vi "Datasocket（上课 主）.vi"() -> ()   [LabVIEW 2017]
uses:
  <vilib>/Analysis/NI_AALBase.lvlib
panel:
  in  "等待时间（毫秒）":u32=10
  out "输出簇":T1
  out "波形图":dbl[](graph)
  in  "停止":bool
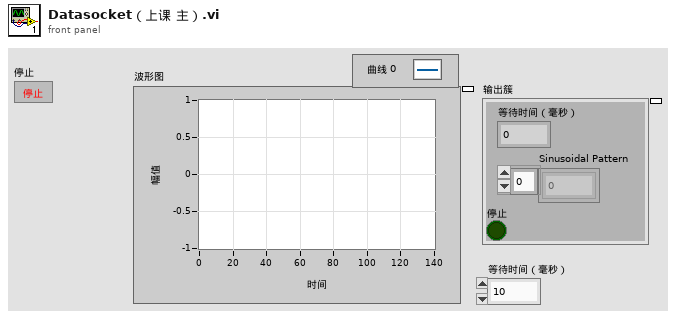
[diagram p1: front panel]
types:
  T1 = cluster{"等待时间（毫秒）":u32, "Sinusoidal Pattern":dbl[], "停止":bool}
  T2 = enum16{"Read", "Write", "ReadWrite", "BufferedRead", "BufferedReadWrite"}
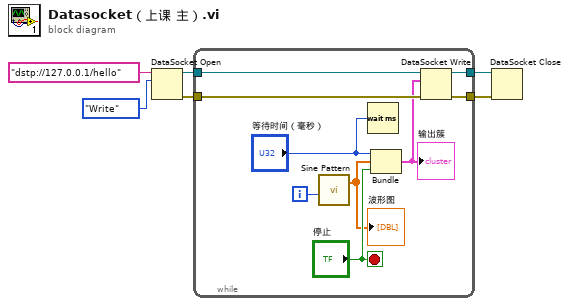
[diagram p0: block diagram]
diagram:
  n1 = DataSocket Open(10:T2."Write" ("模式"), 11:"dstp://127.0.0.1/hello" ("URL")) -> (0:w5:errorcluster, 3:w6:refnum<k13>)  [unwired: 2 in]
  n2 = while {
    tunnel: w6 -> [w11]
    tunnel: w5 -> [w10]
    tunnel: [w8] -> w3
    tunnel: [w7] -> w2
    i -> [w15]
    stop <- "停止" stop-if-true
    n3 = call <vilib>:"Sine Pattern.vi"("phase(degrees)"=w15) -> ("Sinusoidal Pattern"=w13:dbl[])  [unwired: 3 in, 1 out]
    "波形图" <- w13
    n4 = Wait (ms)(milliseconds to wait="等待时间（毫秒）") -> ()  [unwired: 1 out]
    n5 = Bundle("等待时间（毫秒）"="等待时间（毫秒）", "Sinusoidal Pattern"=w13, "停止"="停止") -> (w9:T1)  [unwired: 1 in]
    "输出簇" <- w9
    n6 = DataSocket Write(8:w10, 10:w9, 11:w11) -> (0:w7:errorcluster, 3:w8:refnum<k13>)  [unwired: 1 in, 1 out]
  }
  n7 = DataSocket Close(8:w2, 11:w3) -> ()  [unwired: 1 in, 2 out]
